vi "set valid booleans for data interfaces.vi"(8 "error in":errorcluster, 9 "Channel Specification":T1[](array[typedef]), 10 "vi path":path, 11 "Application in":refnum<vi>) -> (0 "error out":errorcluster)   [LabVIEW 2013, in "FixedChannelTBModuleDecideFeatures.lvclass"]
uses:
  FixedChannelTBModuleDecideFeatures.lvclass
  channel configuration.ctl
  <vilib>/NI/Tag Bus Module Framework/channel/channel classification.ctl
  <vilib>/NI/Tag Bus/tag/Data Type.ctl
  <vilib>/Utility/traverseref.llb/TRef TravTarget.ctl
  <vilib>/Utility/traverseref.llb/VI Scripting - Traverse.lvlib
  <vilib>/NI/Tag Bus Module Framework/channel/TBM channel.lvclass
  <vilib>/NI/Tag Bus/tag/tag descriptor.lvclass
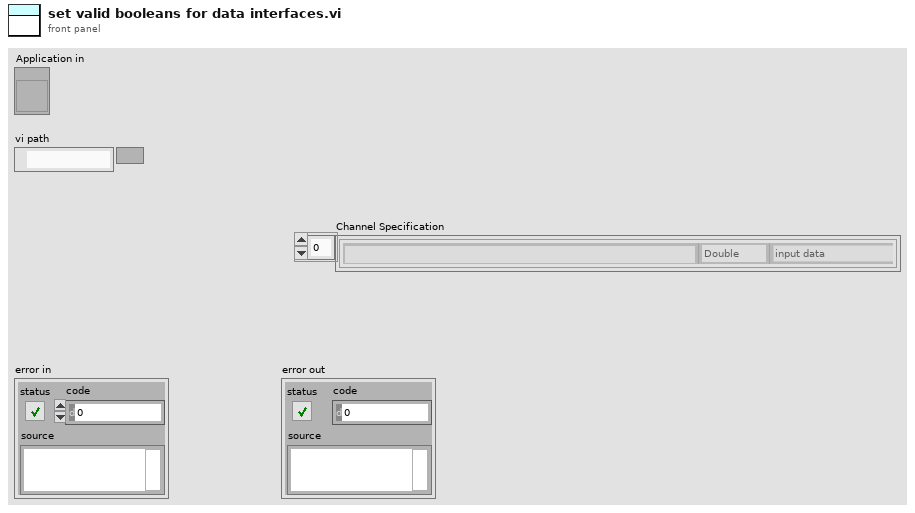
[diagram p1: front panel]
types:
  T1 = typedef "FixedChannelTBModuleDecideFeatures.lvclass/channel configuration.ctl" = cluster{"Name":string, "channel classification":T2, "data type":T3}
  T2 = typedef "TBM channel.lvclass/channel classification.ctl" = enum16{"input data", "output data", "processing parameter", "processing result"}
  T3 = typedef "tag bus.lvlib/tag descriptor.lvclass/Data Type.ctl" = enum16{"Double", "Single", "I64", "I32", "I16", "I8", "U64", "U32", "U16", "U8", "Boolean", "String", "Array of Double", "Array of Single", "Array of I64", "Array of I32", "Array of I16", "Array of I8", "Array of U64", "Array of U32", "Array of U16", "Array of U8", "Array of Boolean", "Array of String"}
  T4 = typedef "TRef TravTarget.ctl" = enum16{"FP", "BD", "Other"}
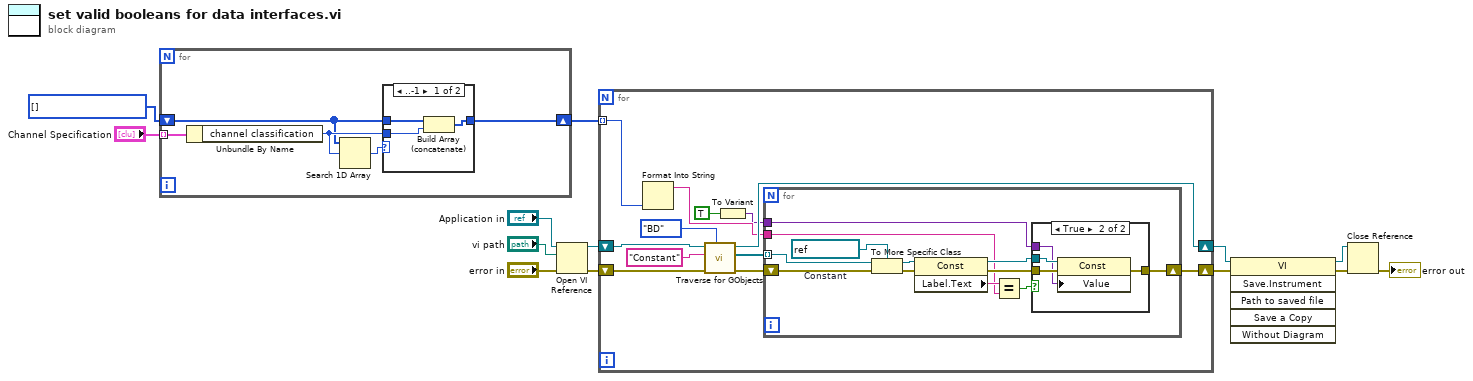
[diagram p0: block diagram]
diagram:
  w3 = T2[] [] items=["input data", "output data", "processing parameter", "processing result"]
  n1 = for {
    tunnel: "Channel Specification" -> [w18] mode=indexing
    shift-right: [w15] -> w2
    shift-left: w3 -> [w14]
    n2 = Unbundle By Name(w18) -> ("channel classification"=w16:T2)
    n3 = Search 1D Array(1D array=w14, element=w16) -> (index of element=w17:i32)  [unwired: 1 in]
    n4 = case shown="..-1" w17 {
      tunnel: w16 -> [w21 _]
      tunnel: [w20 w22] -> w15
      tunnel: w14 -> [w19 w22]
      frame ..-1 {
        n5 = Build Array (concatenate)(w19, w21) -> (w20:T2[])
      }
      frame 0.. {
      }
    }
  }
  n6 = Open VI Reference(application reference (local)="Application in", vi path="vi path", error in (no error)="error in") -> (vi reference=w12:refnum<vi>, error out=w11:errorcluster)  [unwired: 3 in]
  n7 = for {
    shift-right: [w34] -> w13
    shift-left: w11 -> [w28]
    shift-right: [w27] -> w9
    shift-left: w12 -> [w29]
    tunnel: w2 -> [w26] mode=indexing
    n8 = Format Into String(w26) -> (resulting string=w25:string)  [unwired: 3 in, 1 out]
    n9 = call <vilib>:"Traverse for GObjects.vi"("Traverse Target"=TRef_TravTarget."BD", "error in (no error)"=w28, "Class Name"="Constant", "VI Refnum"=w29) -> ("error out"=w32:errorcluster, "References"=w33:refnum<vi>[], "dup VI Refnum"=w27:refnum<vi>)  [unwired: 4 in, 1 out]
    n10 = To Variant(anything=TRUE) -> (Variant=w23:variant)
    n11 = for {
      shift-right: [w39] -> w34
      shift-left: w32 -> [w46]
      tunnel: w33 -> [w45] mode=indexing
      tunnel: w25 -> [w36]
      tunnel: w23 -> [w35]
      w44 = refnum<vi> refnum  # Constant
      n12 = To More Specific Class(target class=w44, reference=w45, error in=w46) -> (specific class reference=w43:refnum<vi>, error out=w42:errorcluster)
      n13 = property class="Const"(reference=w43, error in=w42) -> (reference out=w37:refnum<vi>, error out=w38:errorcluster, "Label.Text"=w41:string)
      n14 = Equal?(x=w41, y=w36) -> (x = y?=w40:bool)
      n15 = case shown="True" w40 {
        tunnel: [w47 w49] -> w39
        tunnel: w38 -> [w47 w51]
        tunnel: w37 -> [_ w50]
        tunnel: w35 -> [_ w48]
        frame False {
        }
        frame True {
          n16 = property class="Const"(reference=w50, error in=w51, "Value"=w48) -> (error out=w49:errorcluster)  [unwired: 1 out]
        }
      }
    }
  }
  n17 = invoke class="VI" method="Save.Instrument"(reference=w9, error in=w13) -> (reference out=w8:refnum<vi>, error out=w10:errorcluster)  [unwired: 4 in, 4 out]
  n18 = Close Reference(reference=w8, error in (no error)=w10) -> (error out=→"error out":errorcluster)
